vi "DHE_DefaultLogicProc.vi"(0 "Database RefNum":T1, 1 "queue":refnum<queue>, 5 "Total Pixels":u32, 7 "Total image Bytes":u32, 9 "tot phys buffers":i32, 11 "error in (no error)":errorcluster, 12 "cont_read":bool, 13 "usc present":bool) -> (15 "error out":errorcluster)   [LabVIEW 2016]
uses:
  DBSHAND/private/vis/DatabaseHand_RefNum.ctl
  Common/public/vis/CMN_FVAR_action.ctl
  DBSHAND/private/vis/DatabaseHand_Element_Get(I32).vi
  DBSHAND/private/vis/DatabaseHand_Element_Get(bool).vi
  DBSHAND/private/vis/DatabaseHand_Element_Get(double).vi
  DBSHAND/private/vis/DatabaseHand_Element_Set(double).vi
  DBSHAND/private/vis/DatabaseHand_Element_Set(bool).vi
  DBSHAND/private/vis/DatabaseHand_Element_Get(U16).vi
  DBSHAND/private/vis/DatabaseHand_Element_Set(U16).vi
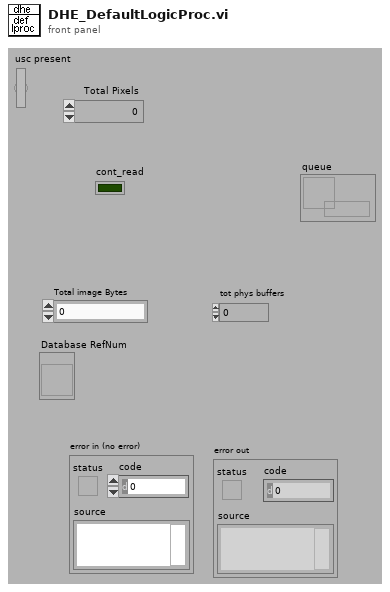
[diagram p1: front panel]
types:
  T1 = typedef "DatabaseHand_RefNum.ctl" = refnum<vi>
  T2 = typedef "CMN_FVAR_action.ctl" = enum16{"read", "write"}
  T3 = cluster{"Name":string, "size (bytes)":u64, "pointer":u64, "Lock":bool}
  T4 = cluster{"pointer":u64, "size":u64, "progress":u32, "status":string}
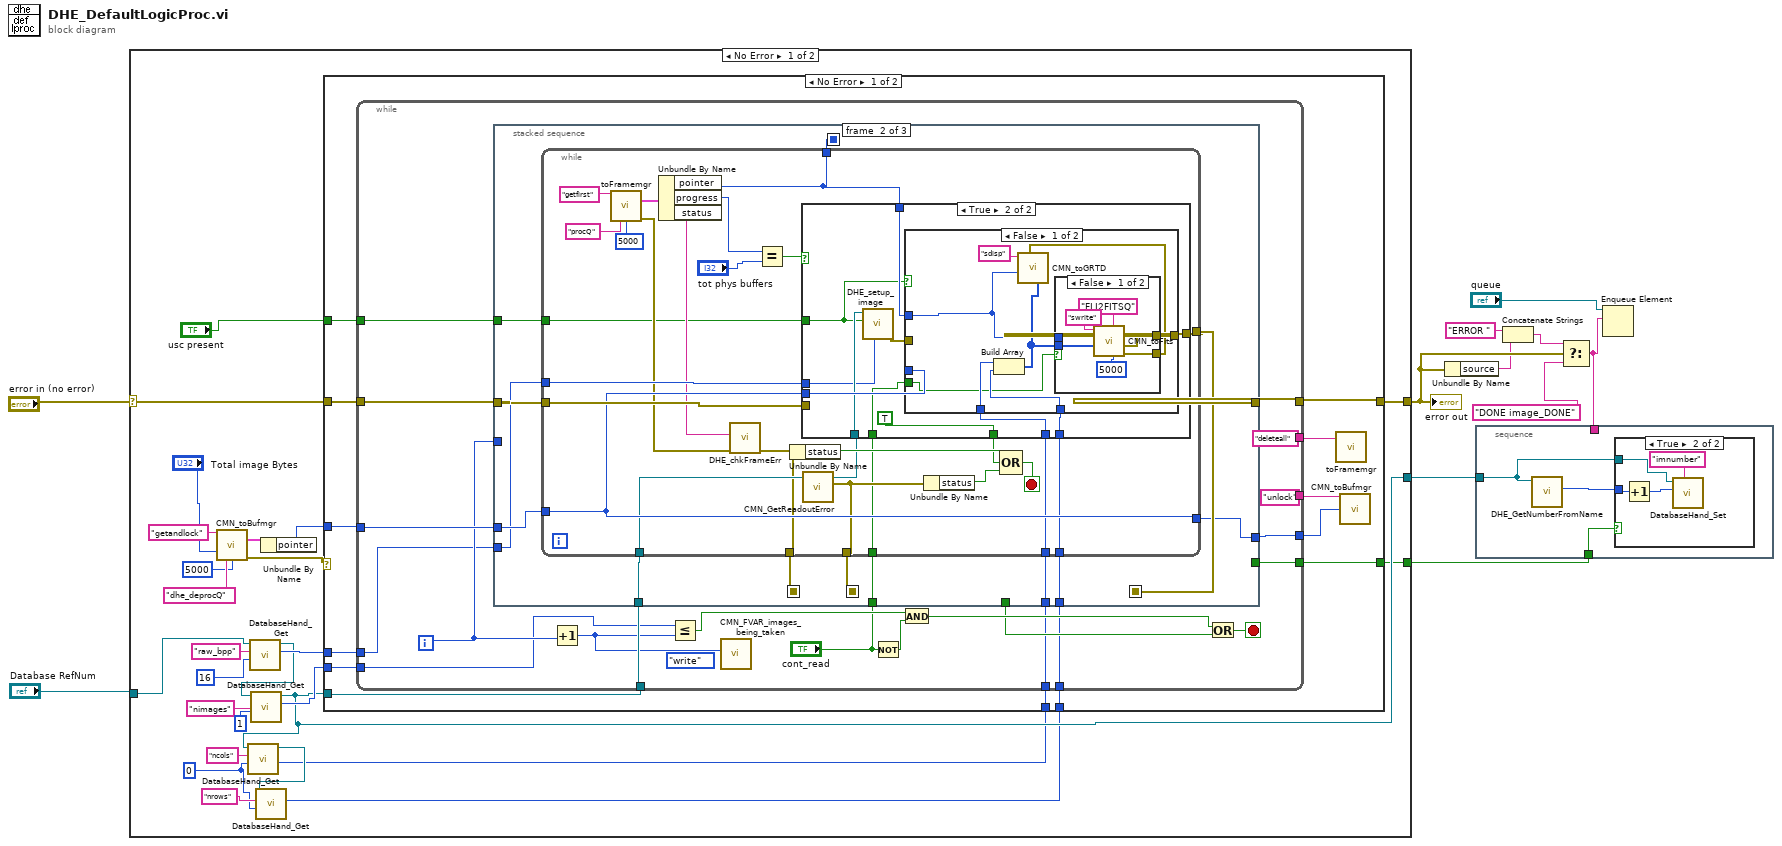
[diagram p0: block diagram]
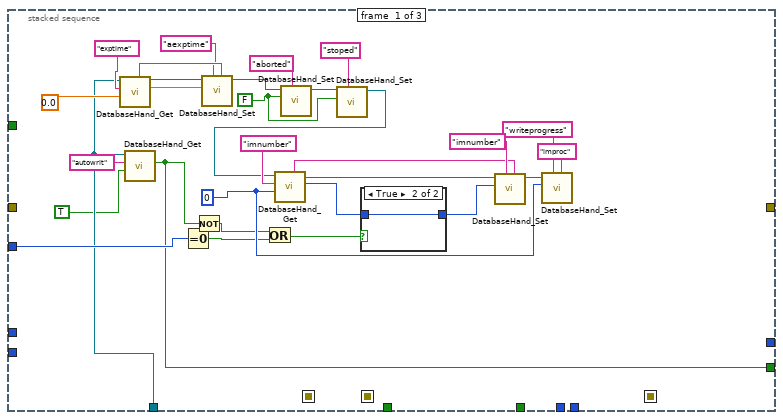
[diagram p3: hidden frame]
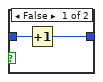
[diagram p4: hidden frame]
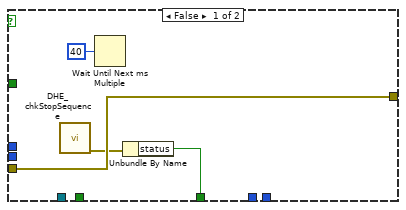
[diagram p5: hidden frame]
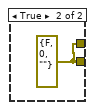
[diagram p6: hidden frame]
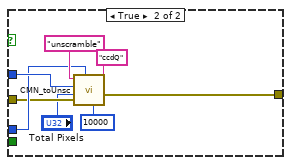
[diagram p7: hidden frame]
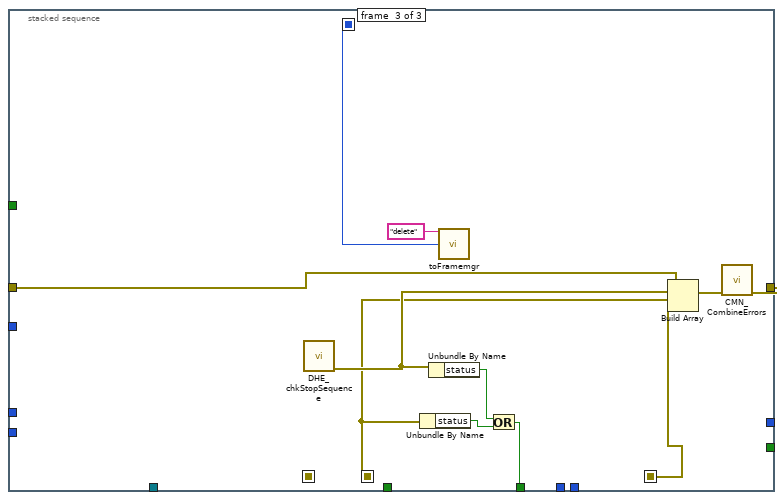
[diagram p8: hidden frame]
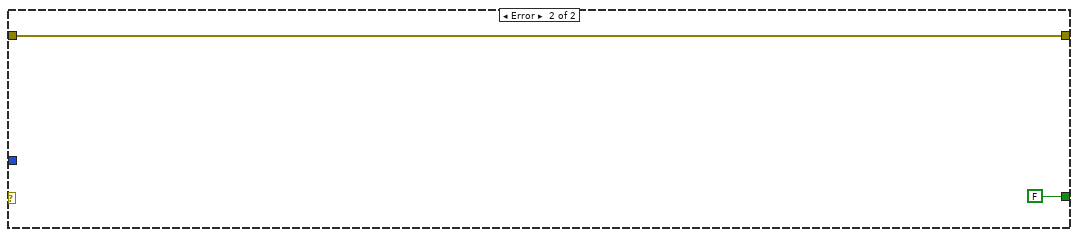
[diagram p9: hidden frame]
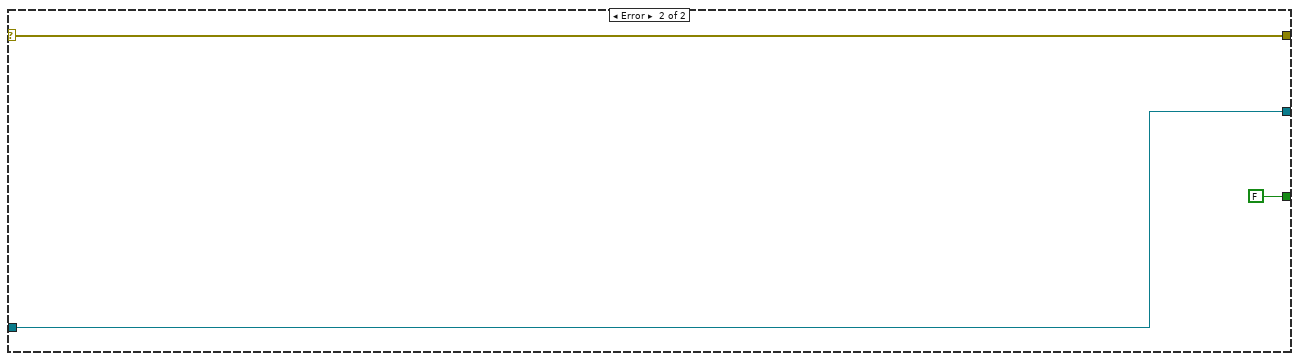
[diagram p10: hidden frame]
diagram:
  n1 = case shown="No Error" "error in (no error)" {
    selector: "error in (no error)" -> [w37 w198]
    tunnel: [w36 w198] -> w5
    tunnel: "Database RefNum" -> [w23 w197]
    tunnel: [w19 w197] -> w3
    tunnel: [w12 FALSE ("value")] -> w1
    frame No Error {
      w15 = 0
      n2 = call "CMN_toBufmgr.vi"("command"="getandlock", "bufsize"="Total image Bytes", "responseQ"="dhe_deprocQ", "ms timeout (-1)"=5000) -> ("buffer"=w33:T3, "error out"=w34:errorcluster)  [unwired: 4 in, 6 out]
      n3 = call-poly "DatabaseHand_Get.vi"("default value"=16, "name"="raw_bpp", "Database RefNum in"=w23) -> ("value"=w26:i32, "Database RefNum out"=w22:T1)  [unwired: 2 in, 5 out]
      n4 = call-poly "DatabaseHand_Get.vi"("default value"=1, "name"="nimages", "Database RefNum in"=w22) -> ("value"=w21:i32, "Database RefNum out"=w19:T1)  [unwired: 2 in, 5 out]
      n5 = call-poly "DatabaseHand_Get.vi"("default value"=w15, "name"="ncols", "Database RefNum in"=w19) -> ("value"=w14:i32, "Database RefNum out"=w18:T1)  [unwired: 2 in, 5 out]
      n6 = call-poly "DatabaseHand_Get.vi"("default value"=w15, "name"="nrows", "Database RefNum in"=w18) -> ("value"=w13:i32)  [unwired: 2 in, 6 out]
      n7 = Unbundle By Name(w33) -> ("pointer"=w32:u64)
      n8 = case shown="No Error" w34 {
        tunnel: w37 -> [w50 w195]
        tunnel: [w49 w195] -> w36
        tunnel: w32 -> [w47 _]
        tunnel: w19 -> [w44 _]
        tunnel: w26 -> [w43 _]
        tunnel: w21 -> [w42 _]
        tunnel: "usc present" -> [w41 _]
        tunnel: w14 -> [w40 _]
        tunnel: w13 -> [w39 _]
        tunnel: [w38 FALSE ("value")] -> w12
        frame No Error {
          n9 = while {
            tunnel: [w71] -> w49
            tunnel: w50 -> [w72]
            tunnel: ["deleteall" ("command")] -> w48
            tunnel: w47 -> [w69]
            tunnel: [w68] -> w46
            tunnel: ["unlock" ("command")] -> w45
            tunnel: w44 -> [w66]
            tunnel: w43 -> [w62]
            tunnel: w42 -> [w60]
            tunnel: w41 -> [w55]
            tunnel: w40 -> [w54]
            tunnel: w39 -> [w53]
            tunnel: [w52] -> w38
            i -> [w65]
            stop <- w61 stop-if-true
            n10 = stacked-sequence {
              seq-local: [_ w117 _] -> [_ _ w188]
              seq-local: [_ w116 _] -> [_ _ w189]
              seq-local: [_ w115 _] -> [_ _ _]
              seq-local: [_ w114 _] -> [_ _ w185]
              tunnel: w72 -> [_ w118 w193]
              tunnel: [_ _ w191] -> w71
              tunnel: w69 -> [_ w113 _]
              tunnel: [_ w112 _] -> w68
              tunnel: w66 -> [w79 w111 _]
              tunnel: w65 -> [w92 _ _]
              tunnel: w62 -> [_ w110 _]
              tunnel: [_ _ w183] -> w56
              tunnel: w55 -> [_ w109 _]
              tunnel: w54 -> [_ w108 _]
              tunnel: w53 -> [_ w107 _]
              tunnel: [w73 _ _] -> w52
              tunnel: "cont_read" -> [_ w106 _]
              frame #0 {
                w83 = FALSE
                w93 = u16 0
                n11 = call-poly "DatabaseHand_Get.vi"("default value"=0.0, "name"="exptime", "Database RefNum in"=w79) -> ("value"=w88:dbl, "Database RefNum out"=w91:T1, "group"=w90:string)  [unwired: 2 in, 4 out]
                n12 = call-poly "DatabaseHand_Get.vi"("default value"=TRUE, "name"="autowrit", "Database RefNum in"=w79) -> ("value"=w73:bool)  [unwired: 2 in, 6 out]
                n13 = Equal To 0?(x=w92) -> (x = 0?=w75:bool)
                n14 = Not(x=w73) -> (.not. x?=w74:bool)
                n15 = call-poly "DatabaseHand_Set.vi"("group"=w90, "name"="aexptime", "value"=w88, "Database RefNum in"=w91) -> ("Database RefNum out"=w86:T1)  [unwired: 4 in, 3 out]
                n16 = Or(x=w74, y=w75) -> (x .or. y?=w76:bool)
                n17 = call-poly "DatabaseHand_Set.vi"("name"="aborted", "value"=w83, "Database RefNum in"=w86) -> ("Database RefNum out"=w85:T1)  [unwired: 5 in, 3 out]
                n18 = call-poly "DatabaseHand_Set.vi"("name"="stoped", "value"=w83, "Database RefNum in"=w85) -> ("Database RefNum out"=w82:T1)  [unwired: 5 in, 3 out]
                n19 = call-poly "DatabaseHand_Get.vi"("default value"=w93, "name"="imnumber", "Database RefNum in"=w82) -> ("value"=w99:u16, "Database RefNum out"=w102:T1, "group"=w100:string)  [unwired: 2 in, 4 out]
                n20 = case shown="True" w76 {
                  tunnel: w99 -> [w104 w105]
                  tunnel: [w103 w105] -> w98
                  frame False {
                    n21 = Increment(x=w104) -> (x+1=w103:u16)
                  }
                  frame True {
                  }
                }
                n22 = call-poly "DatabaseHand_Set.vi"("group"=w100, "name"="imnumber", "value"=w98, "Database RefNum in"=w102) -> ("Database RefNum out"=w96:T1)  [unwired: 4 in, 3 out]
                n23 = call-poly "DatabaseHand_Set.vi"("group"="improc", "name"="writeprogress", "value"=w93, "Database RefNum in"=w96) -> ()  [unwired: 4 in, 4 out]
              }
              frame #1 {
                n24 = while {
                  tunnel: [w127] -> w115
                  tunnel: [w136] -> w116
                  tunnel: [w141] -> w117
                  tunnel: w118 -> [w142]
                  tunnel: [w132] -> w114
                  tunnel: w113 -> [w133]
                  tunnel: [w133] -> w112
                  tunnel: w111 -> [w131]
                  tunnel: w110 -> [w130]
                  tunnel: w109 -> [w122]
                  tunnel: w108 -> [w121]
                  tunnel: w107 -> [w120]
                  tunnel: w106 -> [w119]
                  stop <- w143 stop-if-true
                  n25 = call "toFramemgr.vi"("command"="getfirst", "responseQ"="procQ", "ms timeout (-1)"=5000) -> ("buffer"=w137:T4, "error out"=w129:errorcluster)  [unwired: 6 in, 5 out]
                  n26 = Unbundle By Name(w137) -> ("pointer"=w136:u64, "progress"=w125:u32, "status"=w128:string)
                  n27 = call "DHE_chkFrameErr.vi"("error in"=w129, "frame status"=w128) -> ("error out"=w127:errorcluster)  [unwired: 9 out]
                  n28 = Equal?(x=w125, y="tot phys buffers") -> (x = y?=w134:bool)
                  n29 = Unbundle By Name(w127) -> ("status"=w135:bool)
                  n30 = case shown="True" w134 {
                    tunnel: w142 -> [w146 _]
                    tunnel: [w146 w157] -> w141
                    tunnel: w136 -> [_ w158]
                    tunnel: w133 -> [_ w156]
                    tunnel: w131 -> [_ w155]
                    tunnel: w130 -> [_ w153]
                    tunnel: [w144 TRUE] -> w126
                    tunnel: w122 -> [_ w151]
                    tunnel: w121 -> [_ w150]
                    tunnel: w120 -> [_ w149]
                    tunnel: w119 -> [_ w148]
                    frame False {
                      (unwired) FALSE
                      n31 = call "DHE_chkStopSequence.vi"() -> ("error out"=w145:errorcluster)  [unwired: 11 out]
                      n32 = Wait Until Next ms Multiple(millisecond multiple=u32 40) -> ()  [unwired: 1 out]
                      n33 = Unbundle By Name(w145) -> ("status"=w144:bool)
                    }
                    frame True {
                      n34 = call "DHE_setup_image.vi"("raw bpp"=w153, "usc present"=w151, "Database RefNum in"=w155) -> ("error out"=w154:errorcluster)  [unwired: 2 in, 6 out]
                      n35 = case shown="False" w151 {
                        tunnel: w158 -> [w161 w179]
                        tunnel: [w166 w178] -> w157
                        tunnel: w156 -> [_ w177]
                        tunnel: w154 -> [_ w176]
                        tunnel: w150 -> [w165 _]
                        tunnel: w149 -> [w164 _]
                        tunnel: w148 -> [w159 _]
                        frame False {
                          n36 = Build Array(w165, w164) -> (w162:i32[])
                          n37 = case shown="False" w159 {
                            tunnel: [w168 w174] -> w166
                            tunnel: w162 -> [w171 _]
                            tunnel: w161 -> [w170 _]
                            tunnel: [w169 w174] -> w160
                            frame False {
                              n38 = call "CMN_toFits.vi"("ms timeout (-1)"=5000, "response Q"="FLI2FITSQ", "eleRead"=w171, "location"=w170, "command"="swrite") -> ("error out"=w169:errorcluster, "response"=w168:errorcluster)  [unwired: 3 in, 2 out]
                            }
                            frame True {
                              w174 = errorcluster {"status"=FALSE, "code"=0, "source"=""} ("error out")
                            }
                          }
                          n39 = call "CMN_toGRTD.vi"("Elements"=w162, "error in (no error)"=w160, "location"=w161, "Command"="sdisp") -> ()  [unwired: 4 in, 4 out]
                        }
                        frame True {
                          n40 = call "CMN_toUnsc.vi"("responseQ"="ccdQ", "ms timeout (-1)"=10000, "location 2"=w177, "error in (no error)"=w176, "ele Read"="Total Pixels", "location"=w179, "command"="unscramble") -> ("response"=w178:errorcluster)  [unwired: 2 in, 2 out]
                        }
                      }
                    }
                  }
                  n41 = call "CMN_GetReadoutError.vi"("Database RefNum in"=w131) -> ("readout_error"=w132:errorcluster)  [unwired: 1 in, 9 out]
                  n42 = Unbundle By Name(w132) -> ("status"=w123:bool)
                  n43 = Compound Arithmetic op=OR(w135, w126, w123) -> (w143:bool)
                }
              }
              frame #2 {
                n44 = call "DHE_chkStopSequence.vi"() -> ("error out"=w187:errorcluster)  [unwired: 11 out]
                n45 = Unbundle By Name(w185) -> ("status"=w184:bool)
                n46 = Unbundle By Name(w187) -> ("status"=w186:bool)
                n47 = call "toFramemgr.vi"("command"="delete", "bufpointer"=w189) -> ()  [unwired: 7 in, 7 out]
                n48 = Or(x=w186, y=w184) -> (x .or. y?=w183:bool)
                n49 = Build Array(w193, w187, w185, w188) -> (w192:errorcluster[])
                n50 = call "CMN_CombineErrors.vi"("Errors"=w192) -> ("error out"=w191:errorcluster)  [unwired: 10 out]
              }
            }
            n51 = Increment(x=w65) -> (x+1=w64:i32)
            n52 = Less Or Equal?(x=w60, y=w64) -> (x <= y?=w58:bool)
            n53 = call "CMN_FVAR_images_being_taken.vi"("value in"=w64, "action"=CMN_FVAR_action."write") -> ()  [unwired: 9 out]
            n54 = Not(x="cont_read") -> (.not. x?=w57:bool)
            n55 = And(x=w58, y=w57) -> (x .and. y?=w59:bool)
            n56 = Or(x=w59, y=w56) -> (x .or. y?=w61:bool)
          }
          n57 = call "toFramemgr.vi"("command"=w48) -> ()  [unwired: 8 in, 7 out]
          n58 = call "CMN_toBufmgr.vi"("command"=w45, "bufpointer"=w46) -> ()  [unwired: 6 in, 8 out]
        }
        frame Error {
        }
      }
    }
    frame Error {
    }
  }
  "error out" <- w5
  n59 = Unbundle By Name(w5) -> ("source"=w4:string)
  n60 = Concatenate Strings("ERROR " ("string"), w4) -> (w7:string)
  n61 = Select(t=w7, s=w5, f="DONE image_DONE") -> (s? t:f=w2:string)
  n62 = stacked-sequence {
    tunnel: w3 -> [w201]
    tunnel: w2 -> [_]
    tunnel: w1 -> [w199]
    frame #0 {
      n63 = call "DHE_GetNumberFromName.vi"("Database RefNum in"=w201) -> ("number"=w200:u16)  [unwired: 1 in, 9 out]
      n64 = case shown="True" w199 {
        tunnel: w201 -> [_ w203]
        tunnel: w200 -> [_ w202]
        frame False {
        }
        frame True {
          n65 = Increment(x=w202) -> (x+1=w204:u16)
          n66 = call-poly "DatabaseHand_Set.vi"("name"="imnumber", "value"=w204, "Database RefNum in"=w203) -> ()  [unwired: 5 in, 4 out]
        }
      }
    }
  }
  n67 = Enqueue Element(queue="queue", element=w2) -> ()  [unwired: 1 in, 4 out]
